vi "Create Data Updated User Event.vi"(8 "error in (no error)":errorcluster) -> (0 "error out":errorcluster, 3 "State Update":T1)   [LabVIEW 2015, in "Main Controller Actor.lvclass"]
uses:
  Main Controller Actor.lvclass
  Re-use Libraries/Minimal Actor Framework/Actors/Base Actor/Actor/Update User Event.ctl
  Re-use Libraries/Minimal Actor Framework/Actors/Base Actor/Actor/Actor.lvclass
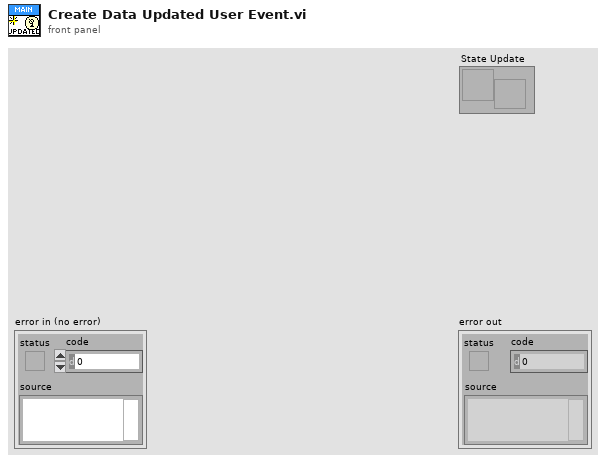
[diagram p1: front panel]
types:
  T1 = typedef "Actor.lvclass/Update User Event.ctl" = refnum<user-event>
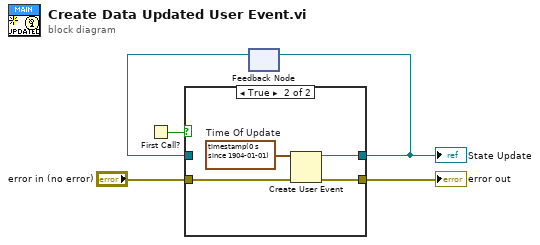
[diagram p0: block diagram]
diagram:
  n1 = First Call?() -> (First Call?: T/F=w3:bool)
  n2 = feedback #1() -> (w2:refnum<user-event>)  [unwired: 1 in]
  n3 = case shown="True" w3 {
    tunnel: "error in (no error)" -> [w7 w9]
    tunnel: [w7 w11] -> w4
    tunnel: [w6 w10] -> w1
    tunnel: w2 -> [w6 _]
    frame False {
    }
    frame True {
      w8 = timestamp(0 s since 1904-01-01)  # Time Of Update
      n4 = Create User Event(user event datatype=w8, error in=w9) -> (user event=w10:refnum<user-event>, error out=w11:errorcluster)
    }
  }
  "error out" <- w4
  "State Update" <- w1
  n5 = feedback-in #1(w1) -> ()
